vi "Brute Force Set Coin.vi"(0 "Input Parsed":T1={"Our Team"=1, "King"={"Set King?"=FALSE, "Min"=0, "Max"=0, "DT Swap Count"=0, "Opp. Swap Count"=0, "DT Pos."={"X"=0, "Y"=0}, "Opp. Pos."={"X"=0, "Y"=0}}, "Board"=[[{"Team"=0, "Occu."=enum."N", "Count"=0}, {"Team"=0, "Occu."=enum."N", "Count"=0}, {"Team"=1, "Occu."=enum."C", "Count"=1}, {"Team"=0, "Occu."=enum."N", "Count"=0}, {"Team"=0, "Occu."=enum."N", "Count"=0}, {"Team"=1, "Occu."=enum."C", "Count"=2}, {"Team"=0, "Occu."=enum."N", "Count"=0}], [{"Team"=0, "Occu."=enum."N", "Count"=0}, {"Team"=0, "Occu."=enum."N", "Count"=0}, {"Team"=0, "Occu."=enum."N", "Count"=0}, {"Team"=0, "Occu."=enum."N", "Count"=0}, {"Team"=1, "Occu."=enum."K", "Count"=0}, {"Team"=2, "Occu."=enum."C", "Count"=1}, {"Team"=1, "Occu."=enum."C", "Count"=1}], [{"Team"=0, "Occu."=enum."N", "Count"=0}, {"Team"=2, "Occu."=enum."C", "Count"=1}, {"Team"=0, "Occu."=enum."N", "Count"=0}, {"Team"=0, "Occu."=enum."N", "Count"=0}, {"Team"=0, "Occu."=enum."N", "Count"=0}, {"Team"=1, "Occu."=enum."C", "Count"=1}, {"Team"=0, "Occu."=enum."N", "Count"=0}], [{"Team"=2, "Occu."=enum."C", "Count"=1}, {"Team"=2, "Occu."=enum."C", "Count"=1}, {"Team"=2, "Occu."=enum."C", "Count"=1}, {"Team"=2, "Occu."=enum."C", "Count"=1}, {"Team"=0, "Occu."=enum."N", "Count"=0}, {"Team"=0, "Occu."=enum."N", "Count"=0}, {"Team"=0, "Occu."=enum."N", "Count"=0}], [{"Team"=2, "Occu."=enum."C", "Count"=1}, {"Team"=0, "Occu."=enum."N", "Count"=0}, {"Team"=1, "Occu."=enum."C", "Count"=1}, {"Team"=0, "Occu."=enum."N", "Count"=0}, {"Team"=1, "Occu."=enum."C", "Count"=1}, {"Team"=0, "Occu."=enum."N", "Count"=0}, {"Team"=0, "Occu."=enum."N", "Count"=0}], [{"Team"=2, "Occu."=enum."C", "Count"=1}, {"Team"=0, "Occu."=enum."N", "Count"=0}, {"Team"=0, "Occu."=enum."N", "Count"=0}, {"Team"=0, "Occu."=enum."N", "Count"=0}, {"Team"=0, "Occu."=enum."N", "Count"=0}, {"Team"=0, "Occu."=enum."N", "Count"=0}, {"Team"=1, "Occu."=enum."C", "Count"=1}], [{"Team"=0, "Occu."=enum."N", "Count"=0}, {"Team"=0, "Occu."=enum."N", "Count"=0}, {"Team"=1, "Occu."=enum."C", "Count"=1}, {"Team"=1, "Occu."=enum."C", "Count"=1}, {"Team"=0, "Occu."=enum."N", "Count"=0}, {"Team"=0, "Occu."=enum."N", "Count"=0}, {"Team"=0, "Occu."=enum."N", "Count"=0}]], "1D Board"=[{"Team"=0, "Occu."=enum."N", "Count"=0}, {"Team"=0, "Occu."=enum."N", "Count"=0}, {"Team"=1, "Occu."=enum."C", "Count"=1}, {"Team"=0, "Occu."=enum."N", "Count"=0}, {"Team"=0, "Occu."=enum."N", "Count"=0}, {"Team"=1, "Occu."=enum."C", "Count"=2}, {"Team"=0, "Occu."=enum."N", "Count"=0}, {"Team"=0, "Occu."=enum."N", "Count"=0}, {"Team"=0, "Occu."=enum."N", "Count"=0}, {"Team"=0, "Occu."=enum."N", "Count"=0}, {"Team"=0, "Occu."=enum."N", "Count"=0}, {"Team"=1, "Occu."=enum."K", "Count"=0}, {"Team"=2, "Occu."=enum."C", "Count"=1}, {"Team"=1, "Occu."=enum."C", "Count"=1}, {"Team"=0, "Occu."=enum."N", "Count"=0}, {"Team"=2, "Occu."=enum."C", "Count"=1}, {"Team"=0, "Occu."=enum."N", "Count"=0}, {"Team"=0, "Occu."=enum."N", "Count"=0}, {"Team"=0, "Occu."=enum."N", "Count"=0}, {"Team"=1, "Occu."=enum."C", "Count"=1}, {"Team"=0, "Occu."=enum."N", "Count"=0}, {"Team"=2, "Occu."=enum."C", "Count"=1}, {"Team"=2, "Occu."=enum."C", "Count"=1}, {"Team"=2, "Occu."=enum."C", "Count"=1}, {"Team"=2, "Occu."=enum."C", "Count"=1}, {"Team"=0, "Occu."=enum."N", "Count"=0}, {"Team"=0, "Occu."=enum."N", "Count"=0}, {"Team"=0, "Occu."=enum."N", "Count"=0}, {"Team"=2, "Occu."=enum."C", "Count"=1}, {"Team"=0, "Occu."=enum."N", "Count"=0}, {"Team"=1, "Occu."=enum."C", "Count"=1}, {"Team"=0, "Occu."=enum."N", "Count"=0}, {"Team"=1, "Occu."=enum."C", "Count"=1}, {"Team"=0, "Occu."=enum."N", "Count"=0}, {"Team"=0, "Occu."=enum."N", "Count"=0}, {"Team"=2, "Occu."=enum."C", "Count"=1}, {"Team"=0, "Occu."=enum."N", "Count"=0}, {"Team"=0, "Occu."=enum."N", "Count"=0}, {"Team"=0, "Occu."=enum."N", "Count"=0}, {"Team"=0, "Occu."=enum."N", "Count"=0}, {"Team"=0, "Occu."=enum."N", "Count"=0}, {"Team"=1, "Occu."=enum."C", "Count"=1}, {"Team"=0, "Occu."=enum."N", "Count"=0}, {"Team"=0, "Occu."=enum."N", "Count"=0}, {"Team"=1, "Occu."=enum."C", "Count"=1}, {"Team"=1, "Occu."=enum."C", "Count"=1}, {"Team"=0, "Occu."=enum."N", "Count"=0}, {"Team"=0, "Occu."=enum."N", "Count"=0}, {"Team"=0, "Occu."=enum."N", "Count"=0}]}, 11 "error in (no error)":errorcluster) -> (4 "Output Text":string="C 34", 15 "error out":errorcluster)   [LabVIEW 2014, in "Dragon Tamers.lvlib"]
uses:
  Dragon Tamers.lvlib
  Typedefs/Input Parsed.ctl
  Typedefs/King.ctl
  Typedefs/Cell Pos.ctl
  Typedefs/Board.ctl
  Typedefs/Board Cell.ctl
  Typedefs/Cell Occupancy.ctl
  <userlib>/_OpenG.lib/array/array.llb/Filter 1D Array with Scalar (I32)__ogtk.vi
panel:
  out "x-y":u32
  in  "Debug?":bool
  in  "Table Control":string[][](table)=[["", "", "", "", "", "", ""], ["", "", "", "", "", "", ""], ["", "", "", "", "", "", ""], ["", "", "", "", "", "", ""], ["", "", "", "", "", "", ""], ["", "", "", "", "", "", ""], ["", "", "", "", "", "", ""]]
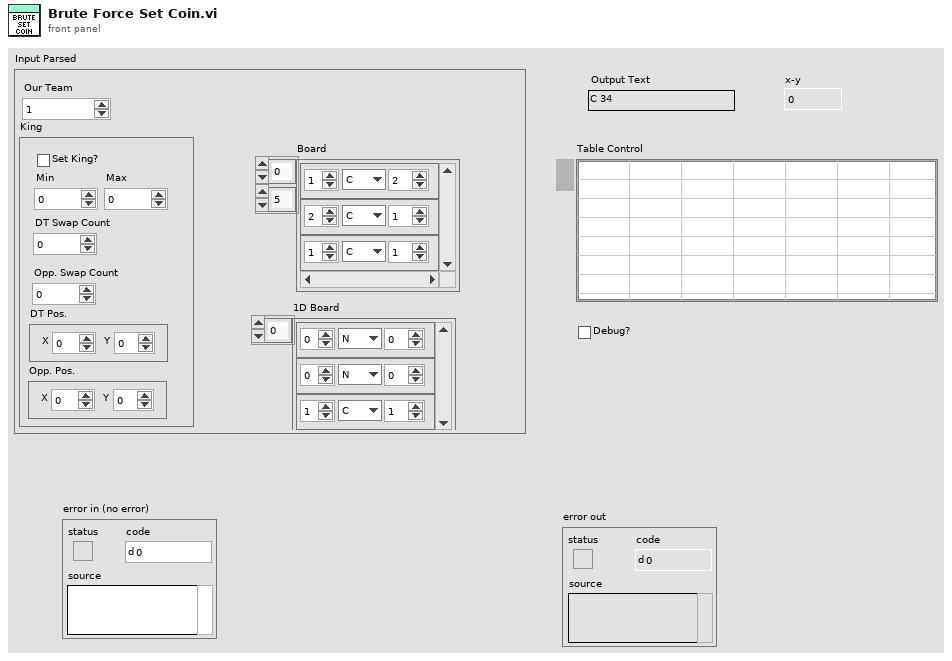
[diagram p1: front panel]
types:
  T1 = typedef "Dragon Tamers.lvlib/Input Parsed.ctl" = cluster{"Our Team":i32, "King":T2, "Board":T4, "1D Board":T5[]}
  T2 = typedef "Dragon Tamers.lvlib/King.ctl" = cluster{"Set King?":bool, "Min":i32, "Max":i32, "DT Swap Count":i32, "Opp. Swap Count":i32, "DT Pos.":T3, "Opp. Pos.":T3}
  T3 = typedef "Dragon Tamers.lvlib/Cell Pos.ctl" = cluster{"X":i32, "Y":i32}
  T4 = typedef "Dragon Tamers.lvlib/Board.ctl" = T5[][]
  T5 = typedef "Dragon Tamers.lvlib/Board Cell.ctl" = cluster{"Team":i32, "Occu.":T6, "Count":i32}
  T6 = typedef "Dragon Tamers.lvlib/Cell Occupancy.ctl" = enum16{"N", "C", "K"}
  T7 = typedef "Dragon Tamers.lvlib/Parsed Board.ctl" = cluster{"DT King":i32, "Opp King":i32, "Count":i32[], "Empty Cells":i32[], "DT Cells":i32[], "Opp Cells":i32[], "DT Team":i32, "Opp. Team":i32}
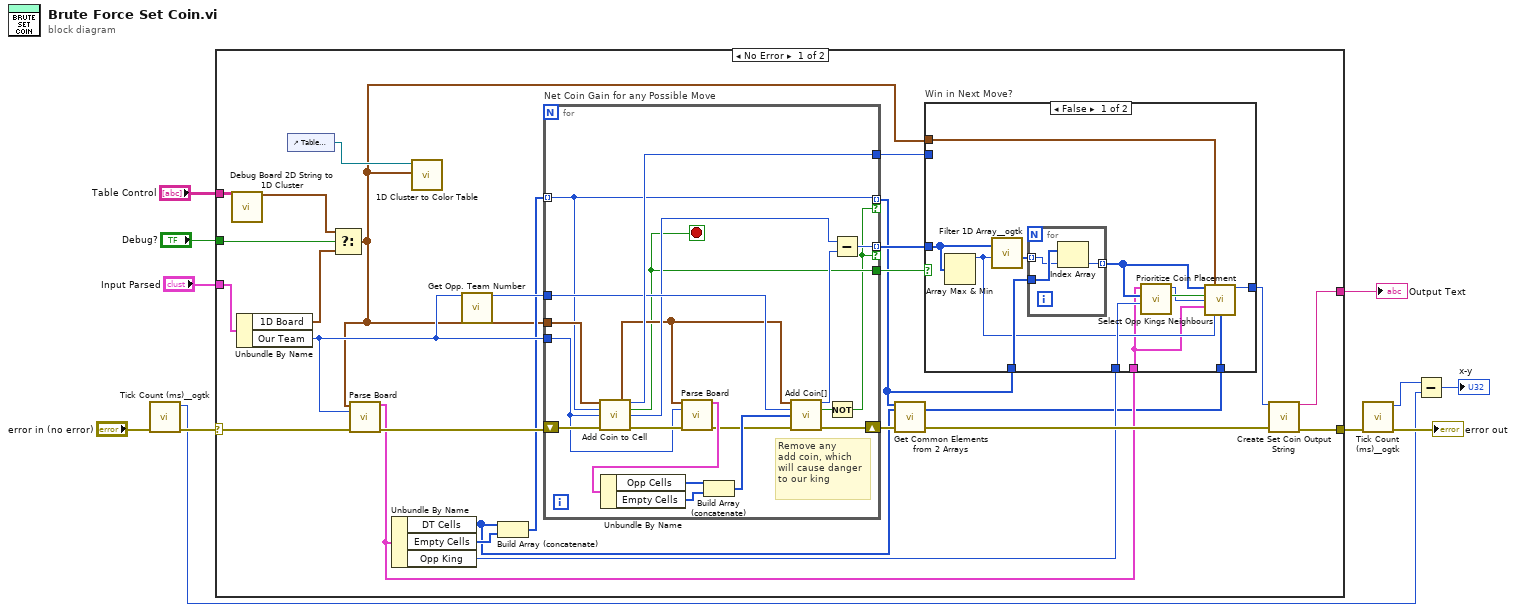
[diagram p0: block diagram]
diagram:
  n1 = call <userlib>:"Tick Count (ms)__ogtk.vi"("error in (no error)"="error in (no error)") -> ("error out"=w6:errorcluster, "millisecond timer value"=w2:u32)  [unwired: 9 in]
  n2 = case shown="No Error" w6 {
    selector: w6 -> [w34 w73]
    tunnel: [w36 w73] -> w5
    tunnel: [w35 _] -> w10
    tunnel: "Input Parsed" -> [w29 _]
    tunnel: "Table Control" -> [w22 _]
    tunnel: "Debug?" -> [w21 _]
    frame No Error {
      n3 = call "Debug Board 2D String to 1D Cluster.vi"("Debug Board 2D String"=w22) -> ("1D Board"=w20:T5[])  [unwired: 14 in]
      n4 = Unbundle By Name(w29) -> ("1D Board"=w19:T5[], "Our Team"=w31:i32)
      n5 = control-ref of="Table Control"() -> (w18:refnum<vi>)
      n6 = Select(t=w20, s=w21, f=w19) -> (s? t:f=w16:T5[])
      n7 = call "Parse Board.vi"("Board Array"=w16, "DT Team #"=w31, "error in (no error)"=w34) -> ("Parsed Board Info"=w26:T7, "error out"=w33:errorcluster)  [unwired: 11 in]
      n8 = Unbundle By Name(w26) -> ("DT Cells"=w14:i32[], "Empty Cells"=w17:i32[], "Opp King"=w27:i32)
      n9 = call "1D Cluster to Color Table.vi"("1D Board"=w16, "Debug Board 2D String Ref"=w18) -> ()  [unwired: 10 in]
      n10 = call "Get Opp. Team Number.vi"("DT Team"=w31) -> ("Opp Team"=w30:i32)  [unwired: 14 in]
      n11 = Build Array (concatenate)(w14, w17) -> (w28:i32[])
      n12 = for "Net Coin Gain for any Possible Move" {
        tunnel: w16 -> [w72]
        tunnel: w28 -> [w54] mode=indexing
        tunnel: w31 -> [w63]
        shift-right: [w69] -> w32
        shift-left: w33 -> [w71]
        tunnel: [w57] -> w15 mode=indexing if=w53
        tunnel: [w70] -> w23
        tunnel: w30 -> [w68]
        tunnel: [w56] -> w24
        tunnel: [w54] -> w13 mode=indexing if=w53
        stop <- w56 stop-if-true
        # "Remove any \nadd coin, which\nwill cause danger\nto our king"
        n13 = call "Add Coin to Cell.vi"("1D Board Array"=w72, "Cell Index"=w54, "Team Number"=w63, "error in (no error)"=w71) -> ("1D Board Array Out"=w65:T5[], "Cell Index"=w70:i32, "Win?"=w56:bool, "Coins Won"=w66:i32, "error out"=w64:errorcluster)  [unwired: 7 in]
        n14 = call "Parse Board.vi"("Board Array"=w65, "DT Team #"=w63, "error in (no error)"=w64) -> ("Parsed Board Info"=w62:T7, "error out"=w58:errorcluster)  [unwired: 11 in]
        n15 = Unbundle By Name(w62) -> ("Opp Cells"=w61:i32[], "Empty Cells"=w60:i32[])
        n16 = Build Array (concatenate)(w61, w60) -> (w59:i32[])
        n17 = call "Add Coin[].vi"("1D Board"=w65, "Team Number"=w68, "Cell Index[]"=w59, "error in (no error)"=w58) -> ("Max Coin Wins"=w67:i32, "Win?"=w55:bool, "error out"=w69:errorcluster)  [unwired: 8 in, 1 out]
        n18 = Not(x=w55) -> (.not. x?=w53:bool)
        n19 = Subtract(x=w66, y=w67) -> (x-y=w57:i32)
      }
      n20 = call "Get Common Elements from 2 Arrays.vi"("Array 1"=w13, "Array 2"=w14) -> ("Common Array"=w12:i32[])  [unwired: 15 in, 2 out]
      n21 = case "Win in Next Move?" shown="False" w24 {
        tunnel: w15 -> [w48 _]
        tunnel: w13 -> [w47 _]
        tunnel: w27 -> [w45 _]
        tunnel: w26 -> [w38 _]
        tunnel: [w42 w52] -> w25
        tunnel: w23 -> [_ w52]
        tunnel: w16 -> [w39 _]
        tunnel: w12 -> [w37 _]
        frame False {
          n22 = Array Max & Min(array=w48) -> (max value=w40:i32)  [unwired: 3 out]
          n23 = call-poly <userlib>:"Filter 1D Array__ogtk.vi"("items to filter"=w40, "array"=w48) -> ("filtered item indices"=w46:i32[])  [unwired: 4 in, 1 out]
          n24 = for {
            tunnel: w46 -> [w50] mode=indexing
            tunnel: w47 -> [w51]
            tunnel: [w49] -> w41 mode=indexing
            n25 = Index Array(array=w51, index=w50) -> (element=w49:i32)
          }
          n26 = call "Select Opp Kings Neighbours.vi"("Opp King Cell Index"=w45, "Candidate Cells"=w41, "Parsed Board"=w38) -> ("Moving to Opp. King's Neighbour?"=w44:bool, "Selected Cell"=w43:i32)  [unwired: 7 in]
          n27 = call "Prioritize Coin Placement.vi"("Candidate Cells"=w41, "Board Array"=w39, "Moving to Opp. King's Neighbour?"=w44, "Move Index"=w43, "Parsed Board Info"=w38, "Net Cell Gain"=w40, "Danger Free DT Cells"=w37) -> ("Move Index"=w42:i32)  [unwired: 7 in, 1 out]
        }
        frame True {
          # "Do the winning move"
        }
      }
      n28 = call "Create Set Coin Output String.vi"("Cell Index"=w25, "error in (no error)"=w32) -> ("Output Text"=w35:string, "error out"=w36:errorcluster)  [unwired: 12 in]
    }
    frame Error {
    }
  }
  "Output Text" <- w10
  n29 = call <userlib>:"Tick Count (ms)__ogtk.vi"("error in (no error)"=w5) -> ("error out"=→"error out":errorcluster, "millisecond timer value"=w3:u32)  [unwired: 9 in]
  n30 = Subtract(x=w3, y=w2) -> (x-y=→"x-y":u32)
